vi "Camera Tester - No VA.vi"() -> ()   [LabVIEW 2020]
uses:
  <vilib>/vision/driver/IMAQdx.llb/IMAQdx Buffer Number Mode.ctl
  <vilib>/vision/driver/NI_Vision_Acquisition_Software.lvlib
  <vilib>/vision/NI_Vision_Development_Module.lvlib
panel:
  out "Time Elapsed (msec)":dbl
  out "Distance (mm)":dbl format="%.2f"
  in  "Camera Name":refnum<k21> caption="IMAQdx Session"
  out "Acquisition Frame Rate":dbl
  out "Buffer Number":u32
  out "Image":T1(plugin-control)
  in  "Stop":bool
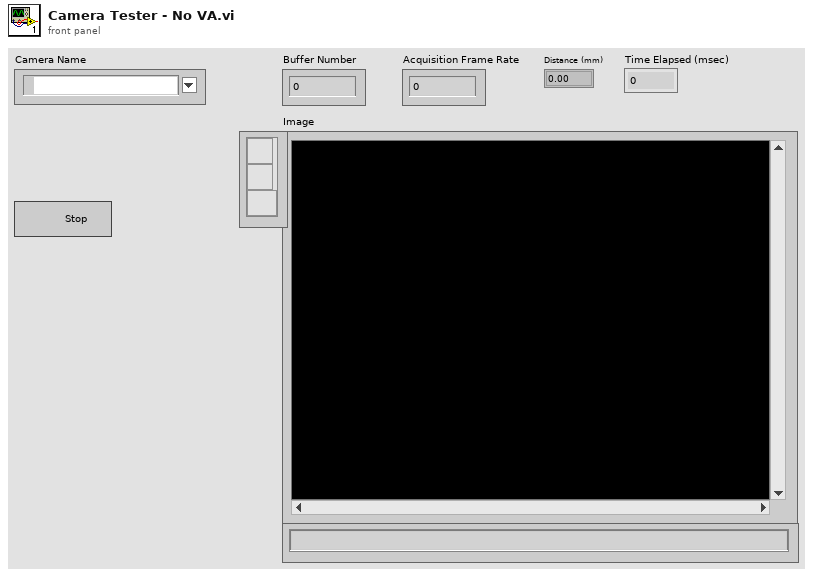
[diagram p1: front panel]
types:
  T1 = typedef "IMAQ Image.ctl" = refnum<image>
  T2 = typedef "IMAQdx.ctl" = refnum<k21>
  T3 = cluster{"Contrast":i32, "Filter width":i32, "Steepness":i32, "Subsampling Ratio":u32, "Show Search Area":bool, "Show Search Lines":bool, "Show Edges Found":bool, "Show Result":bool}
  T4 = typedef "NI_Vision_Acquisition_Software.lvlib/IMAQdx Buffer Number Mode.ctl" = enum32{"Next", "Last", "Buffer Number", "Every", "Last New"}
  T5 = cluster{"Global Rectangle":i32[], "Contours":cluster{"Contour Type":u32, "ROI Type":u32, "Points":i32[]}[]}
  T6 = typedef "IMAQ Rectangle" = cluster{"Left":i32, "Top":i32, "Right":i32, "Bottom":i32, "Rotation":dbl}
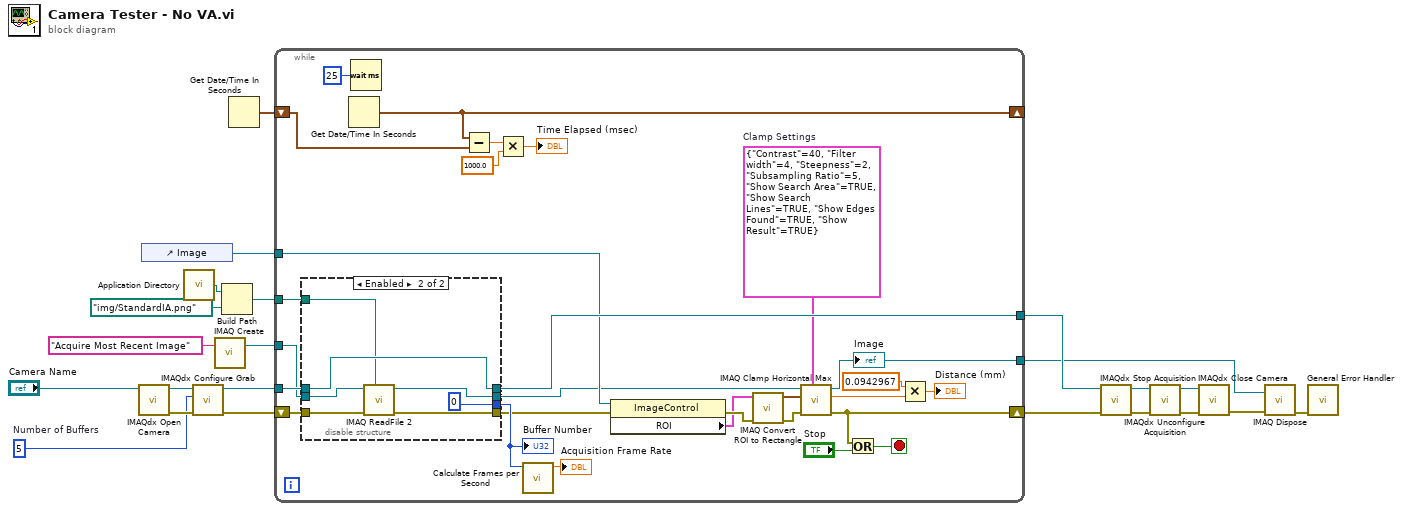
[diagram p0: block diagram]
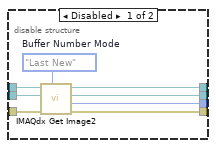
[diagram p2: hidden frame]
diagram:
  w12 = u32 5  # Number of Buffers
  n1 = call <vilib>:"IMAQdx Open Camera.vi"("Session In"="Camera Name") -> ("error out"=w14:errorcluster, "Session Out"=w15:T2)  [unwired: 2 in, 7 out]
  n2 = control-ref of="Image"() -> (w5:refnum<vi>)
  n3 = call <vilib>:"Application Directory.vi"() -> ("Application Directory"=w2:path)
  n4 = call <vilib>:"IMAQdx Configure Grab.vi"("error in"=w14, "Number of Buffers"=w12, "Session In"=w15) -> ("error out"=w10:errorcluster, "Session Out"=w11:T2)  [unwired: 7 in]
  n5 = call "IMAQ Create"("Image Name"="Acquire Most Recent Image") -> ("New Image"=w9:T1)  [unwired: 3 in, 2 out]
  n6 = Build Path(base path=w2, name or relative path=path "img/StandardIA.png") -> (appended path=w3:path)
  n7 = Get Date/Time In Seconds() -> (seconds since 1Jan1904=w4:timestamp)
  n8 = while {
    shift-right: [w37] -> w7
    shift-left: w10 -> [w46]
    tunnel: w9 -> [w45]
    tunnel: [w32] -> w6
    tunnel: w11 -> [w47]
    tunnel: [w44] -> w8
    tunnel: w5 -> [w41]
    shift-right: [w31] -> _
    shift-left: w4 -> [w30]
    tunnel: w3 -> [w29]
    stop <- w43 stop-if-true
    w33 = T3 {"Contrast"=40, "Filter width"=4, "Steepness"=2, "Subsampling Ratio"=5, "Show Search Area"=TRUE, "Show Search Lines"=TRUE, "Show Edges Found"=TRUE, "Show Result"=TRUE}  # Clamp Settings
    n9 = disable-structure shown="Enabled" {
      disable-tunnel: [w57 u32 0 ("Buffer Number")] -> w49
      disable-tunnel: w47 -> [w56 w65]
      disable-tunnel: w46 -> [w55 w63]
      disable-tunnel: w45 -> [w54 w59]
      disable-tunnel: [w53 w65] -> w44
      disable-tunnel: [w52 w62] -> w40
      disable-tunnel: [w51 w61] -> w34
      disable-tunnel: w29 -> [_ w60]
      frame Disabled {
        w58 = IMAQdx_Buffer_Number_Mode."Last New"  # Buffer Number Mode
        n10 = call <vilib>:"IMAQdx Get Image2.vi"("Buffer Number Mode (Next)"=w58, "error in"=w55, "Image In"=w54, "Session In"=w56) -> ("error out"=w52:errorcluster, "Buffer Number Out"=w57:u32, "Image Out"=w51:T1, "Session Out"=w53:T2)  [unwired: 4 in]
      }
      frame Enabled {
        n11 = call "IMAQ ReadFile 2"("File Path"=w60, "error in (no error)"=w63, "Image"=w59) -> ("error out"=w62:errorcluster, "Image Out"=w61:T1)  [unwired: 4 in, 3 out]
      }
    }
    "Buffer Number" <- w49
    n12 = Get Date/Time In Seconds() -> (seconds since 1Jan1904=w31:timestamp)
    n13 = Wait (ms)(milliseconds to wait=u32 25) -> ()  [unwired: 1 out]
    n14 = Subtract(x=w31, y=w30) -> (x-y=w28:dbl)
    n15 = Multiply(x=w28, y=1000.0) -> (x*y=→"Time Elapsed (msec)":dbl)
    n16 = call <vilib>:"Calculate Frames per Second.vi"("Buffer Number"=w49) -> ("Acquired Frames/s"=→"Acquisition Frame Rate":dbl)  [unwired: 8 in, 2 out]
    n17 = property class="ImageControl"(reference=w41, error in=w40) -> (error out=w39:errorcluster, "ROI"=w36:T5)  [unwired: 1 out]
    n18 = call "IMAQ Convert ROI to Rectangle"("error in (no error)"=w39, "ROI Descriptor"=w36) -> ("error out"=w38:errorcluster, "Rectangle"=w35:T6)  [unwired: 7 in]
    n19 = call "IMAQ Clamp Horizontal Max"("Settings"=w33, "error in (no error)"=w38, "Rectangle"=w35, "Image"=w34) -> ("error out"=w37:errorcluster, "Distance"=w24:sgl, "Image Out"=w32:T1)  [unwired: 3 in, 2 out]
    "Image" <- w32
    n20 = Or(x=w37, y="Stop") -> (x .or. y?=w43:bool)
    n21 = Multiply(x=0.0942967, y=w24) -> (x*y=→"Distance (mm)":dbl)
  }
  n22 = call <vilib>:"IMAQdx Stop Acquisition.vi"("error in"=w7, "Session In"=w8) -> ("error out"=w19:errorcluster, "Session Out"=w20:T2)  [unwired: 8 out]
  n23 = call <vilib>:"IMAQdx Unconfigure Acquisition.vi"("error in"=w19, "Session In"=w20) -> ("error out"=w22:errorcluster, "Session Out"=w21:T2)  [unwired: 8 out]
  n24 = call <vilib>:"IMAQdx Close Camera.vi"("error in"=w22, "Session In"=w21) -> ("error out"=w18:errorcluster)  [unwired: 9 out]
  n25 = call "IMAQ Dispose"("Image"=w6, "error in (no error)"=w18) -> ("error out"=w17:errorcluster)  [unwired: 4 in]
  n26 = call <vilib>:"General Error Handler.vi"("error in (no error)"=w17) -> ()  [unwired: 2 in, 13 out]
